vi "Update RTM.vi"(8 "error in (no error)":errorcluster, 11 "TopLevel In":T1) -> (0 "error out":errorcluster)   [LabVIEW 2011]
uses:
  Controls/Top Level Control.ctl
  <vilib>/NI/AMC/Message Queue.ctl
  <vilib>/NI/AMC/Message.ctl
  <vilib>/NI/Tools/Keyed Array/KeyedArray.ctl
  Controls/ListBox Test Record.ctl
  Controls/DVR of CSV Tests Data.ctl
  Controls/CSVs Tests Data.ctl
  Controls/Test Column Data.ctl
  Controls/Options DVR.ctl
  Controls/Options.ctl
  <vilib>/NI/Tools/Keyed Array/Tools_KeyedArray.lvlib
  <vilib>/NI/AMC/AMC.lvlib
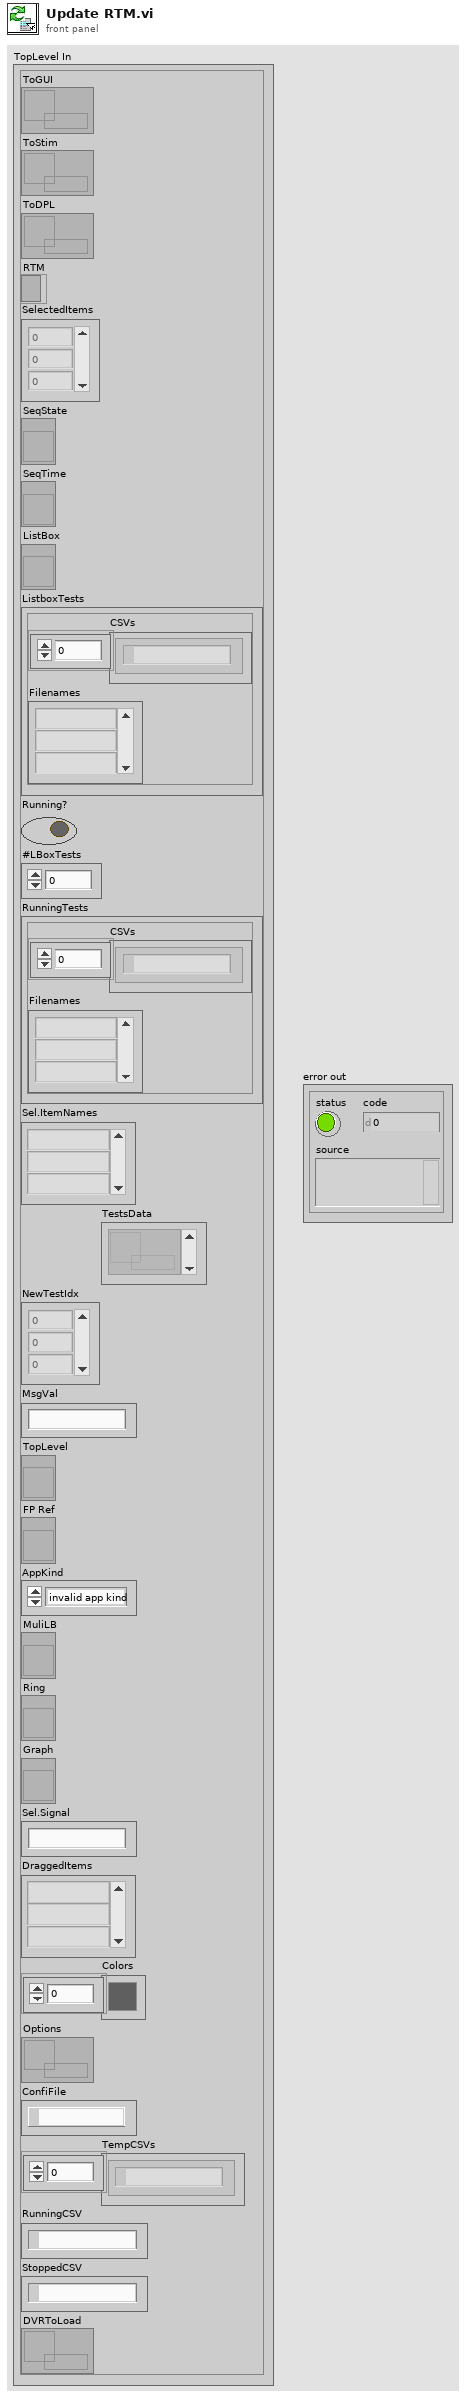
[diagram p1: front panel]
types:
  T1 = typedef "Top Level Control.ctl" = cluster{"ToGUI":T2, "ToStim":T2, "ToDPL":T2, "RTM":refnum<k9>, "SelectedItems":i32[], "SeqState":refnum<vi>, "SeqTime":refnum<vi>, "ListBox":refnum<vi>, "ListboxTests":T3, "Running?":bool, "#LBoxTests":i32, "RunningTests":T3, "Sel.ItemNames":string[], "TestsData":T4[], "NewTestIdx":i32[], "MsgVal":string, "TopLevel":refnum<vi>, "FP Ref":refnum<vi>, "AppKind":enum32{"invalid app kind", "Development System", "Run Time System", "Student Edition", "Embedded LabVIEW", "Evaluation", "Custom"}, "MuliLB":refnum<vi>, "Ring":refnum<vi>, "Graph":refnum<vi>, "Sel.Signal":string, "DraggedItems":string[], "Colors":u32[], "Options":T5, "ConfiFile":path, "TempCSVs":path[], "RunningCSV":path, "StoppedCSV":path, "DVRToLoad":T4}
  T2 = typedef "AMC.lvlib/Message Queue.ctl" = refnum<queue>
  T3 = typedef "ListBox Test Record.ctl" = cluster{"CSVs":path[], "Filenames":string[]}
  T4 = typedef "DVR of CSV Tests Data.ctl" = refnum<data-value>
  T5 = typedef "Options DVR.ctl" = refnum<data-value>
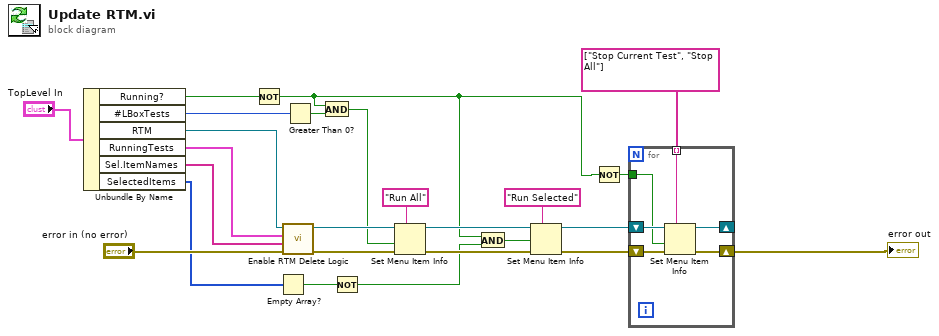
[diagram p0: block diagram]
diagram:
  n1 = Unbundle By Name("TopLevel In") -> ("Running?"=w12:bool, "#LBoxTests"=w19:i32, "RTM"=w25:refnum<k9>, "RunningTests"=w2:T3, "Sel.ItemNames"=w1:string[], "SelectedItems"=w3:i32[])
  n2 = Not(x=w12) -> (.not. x?=w7:bool)
  n3 = Empty Array?(array=w3) -> (empty?=w5:bool)
  n4 = call "Enable RTM Delete Logic.vi"("error in (no error)"="error in (no error)", "Sel.ItemNames"=w1, "Running Tests"=w2, "Menu in"=w25) -> ("error out"=w22:errorcluster, "Menu out"=w21:refnum<k9>)  [unwired: 6 in]
  n5 = Greater Than 0?(x=w19) -> (x > 0?=w18:bool)
  n6 = And(x=w7, y=w18) -> (x .and. y?=w17:bool)
  n7 = Not(x=w5) -> (.not. x?=w4:bool)
  n8 = Set Menu Item Info(7:"Run All" ("item tag"), 8:w22, 9:w17, 11:w21) -> (0:w15:errorcluster, 3:w14:refnum<k9>)  [unwired: 3 in]
  n9 = And(x=w7, y=w4) -> (x .and. y?=w13:bool)
  n10 = Set Menu Item Info(7:"Run Selected" ("item tag"), 8:w15, 9:w13, 11:w14) -> (0:w10:errorcluster, 3:w11:refnum<k9>)  [unwired: 3 in]
  n11 = Not(x=w7) -> (.not. x?=w8:bool)
  n12 = for {
    shift-right: [w28] -> _
    shift-left: w11 -> [w30]
    shift-right: [w29] -> w6
    shift-left: w10 -> [w31]
    tunnel: string[] ["Stop Current Test", "Stop All"] -> [w27] mode=indexing
    tunnel: w8 -> [w26]
    n13 = Set Menu Item Info(7:w27, 8:w31, 9:w26, 11:w30) -> (0:w29:errorcluster, 3:w28:refnum<k9>)  [unwired: 3 in]
  }
  "error out" <- w6
